vi "Autotest_Instr.vi"(8 "error in (no error)":errorcluster caption="entrée d'erreur (pas d'erreur)", 11 "Class Instrument Power_Supply en entrée":refnum<class "Class Instrument Power_Supply.lvclass">) -> (0 "error out":errorcluster caption="sortie d'erreur", 3 "Class Instrument Power_Supply en sortie":refnum<class "Class Instrument Power_Supply.lvclass">)   [LabVIEW 2020, in "Library Instrument & Equipement.lvlib" / "Library Instruments.lvlib" / "Class Instrument Power_Supply.lvclass"]
uses:
  Class Instrument Power_Supply.lvclass
  C:/Users/ngarcin/OneDrive - Altyor/Standard TB/Class/Instrument/Instrument (Default)/Class Instrument (Default).lvclass
  Class Instrument Power_Supply.lvclass/Class Instrument Power_Supply.ctl
  Instrument (Default)/Class Instrument (Default).lvclass
  Power_Supply/Power_Supply (Default)/Power_Supply (Default).lvclass
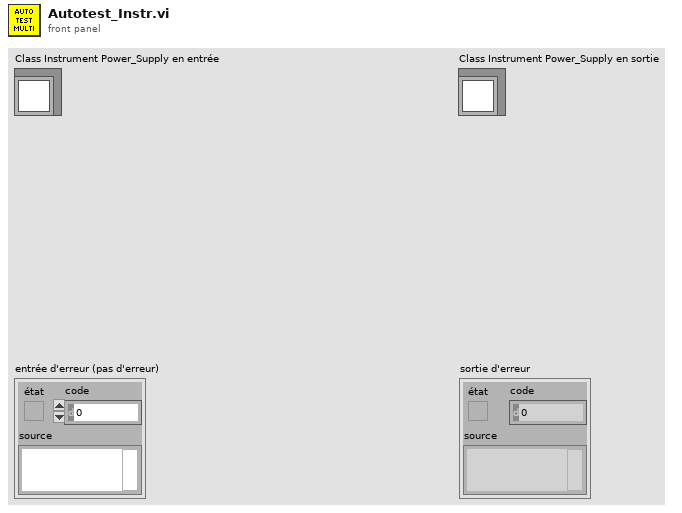
[diagram p1: front panel]
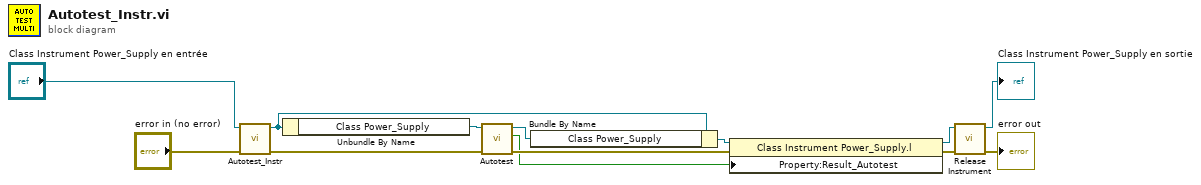
[diagram p0: block diagram]
diagram:
  n1 = call-parent "Autotest_Instr.vi"("error in (no error)"="error in (no error)", "Class Instrument (Default) en entrée"="Class Instrument Power_Supply en entrée") -> ("error out"=w10:errorcluster, "Class Instrument (Default) en sortie"=w11:refnum<class "Class Instrument Power_Supply.lvclass">)  [unwired: 8 in]
  n2 = Unbundle By Name(w11) -> ("Class Power_Supply"=w9:refnum<class "Power_Supply (Default).lvclass">)
  n3 = call-dynamic "Autotest.vi"("error in (no error)"=w10, "Power_Supply (Default) en entrée"=w9) -> ("error out"=w6:errorcluster, "Autotest Ok ?"=w5:bool, "Power_Supply (Default) en sortie"=w8:refnum<class "Power_Supply (Default).lvclass">)  [unwired: 7 in]
  n4 = Bundle By Name(cluster=w11, "Class Power_Supply"=w8) -> (w7:refnum<class "Class Instrument Power_Supply.lvclass">)
  n5 = property class="Class Instrument Power_Supply.l"(reference=w7, error in=w6, "Property:Result_Autotest"=w5) -> (reference out=w2:refnum<class "Class Instrument Power_Supply.lvclass">, error out=w4:errorcluster)
  n6 = call-dynamic "Release Instrument.vi"("error in (no error)"=w4, "Class Instrument (Default) en entrée"=w2) -> ("error out"=→"error out":errorcluster, "Class Instrument (Default) en sortie"=→"Class Instrument Power_Supply en sortie":refnum<class "Class Instrument Power_Supply.lvclass">)  [unwired: 8 in]
